vi "GV preline gate.vi"() -> ()   [LabVIEW 2017]
panel:
  out "Preline gate":bool
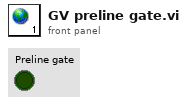
[diagram p1: front panel]
diagram:
